vi "Container To Label.vi"(1 "ActiveX Container":refnum<vi>) -> (0 "Label":refnum<k24>)   [LabVIEW 2020, in "Dot Net UI Controls.lvlib"]
uses:
  Dot Net UI Controls.lvlib
  System.Windows.Forms
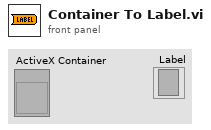
[diagram p1: front panel]
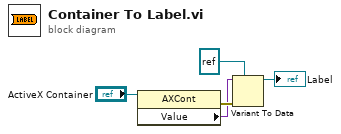
[diagram p0: block diagram]
diagram:
  n1 = property class="AXCont"(reference="ActiveX Container") -> (error out=w5:errorcluster, "Value"=w3:variant)  [unwired: 1 in, 1 out]
  n2 = Variant To Data(error in=w5, type=refnum<k24> refnum ("label ref"), Variant=w3) -> (data=→"Label":refnum<k24>)  [unwired: 1 out]
